vi "Pass State Machine.vi"   [LabVIEW 2013]
uses:
  typedefs/fg_typedef.ctl
  typedefs/subStates.ctl
  typedefs/DevRef Type.ctl
panel:
  # "A State Machine to Handle Passing"
types:
  T1 = typedef "subStates.ctl" = enum16{"null", "wait", "driver control", "auto", "manual override", "hold position", "rotate", "pickup", "pass", "load", "goto shoot", "shoot high goal", "shoot low goal", "cancel arm", "cancel shooter", "end"}
  T2 = typedef "fg_typedef.ctl" = enum16{"Get", "Set"}
  T3 = typedef "DevRef Type.ctl" = enum16{"Shooter Solenoid", "Latch Solenoid", "Right Up Sensor", "Right Down Sensor", "Hold Sensor", "2 Ball Switch", "Arm Encoder"}
  T4 = typedef "WPI_DigitalInputDevRef.ctl" = cluster{"DevStatus":errorcluster, "DIO Channel":T5, "Digital Module":T6}
  T5 = typedef "FPGA_DIOChannel.ctl" = enum8{"DIO 1", "DIO 2", "DIO 3", "DIO 4", "DIO 5", "DIO 6", "DIO 7", "DIO 8", "DIO 9", "DIO 10", "DIO 11", "DIO 12", "DIO 13", "DIO 14", "Invalid"}
  T6 = typedef "FPGA_TypedefDigitalModule.ctl" = enum16{"Digital Module 1", "Digital Module 2"}
  T7 = typedef "WPI_EncoderDevRef.ctl" = cluster{"DevStatus":errorcluster, "EncoderIndex":T8, "CounterIndex":T9, "DistancePerCount":dbl, "Decoding Type":T10}
  T8 = typedef "FPGA_EncoderIdx.ctl" = enum8{"Enc 0", "Enc 1", "Enc 2", "Enc 3", "Invalid"}
  T9 = typedef "FPGA_CounterCtrSystemIndex.ctl" = enum8{"Ctr 0", "Ctr 1", "Ctr 2", "Ctr 3", "Ctr 4", "Ctr 5", "Ctr 6", "Ctr 7", "Invalid"}
  T10 = typedef "WPI_EncoderType.ctl" = enum16{"1x", "2x", "4x"}
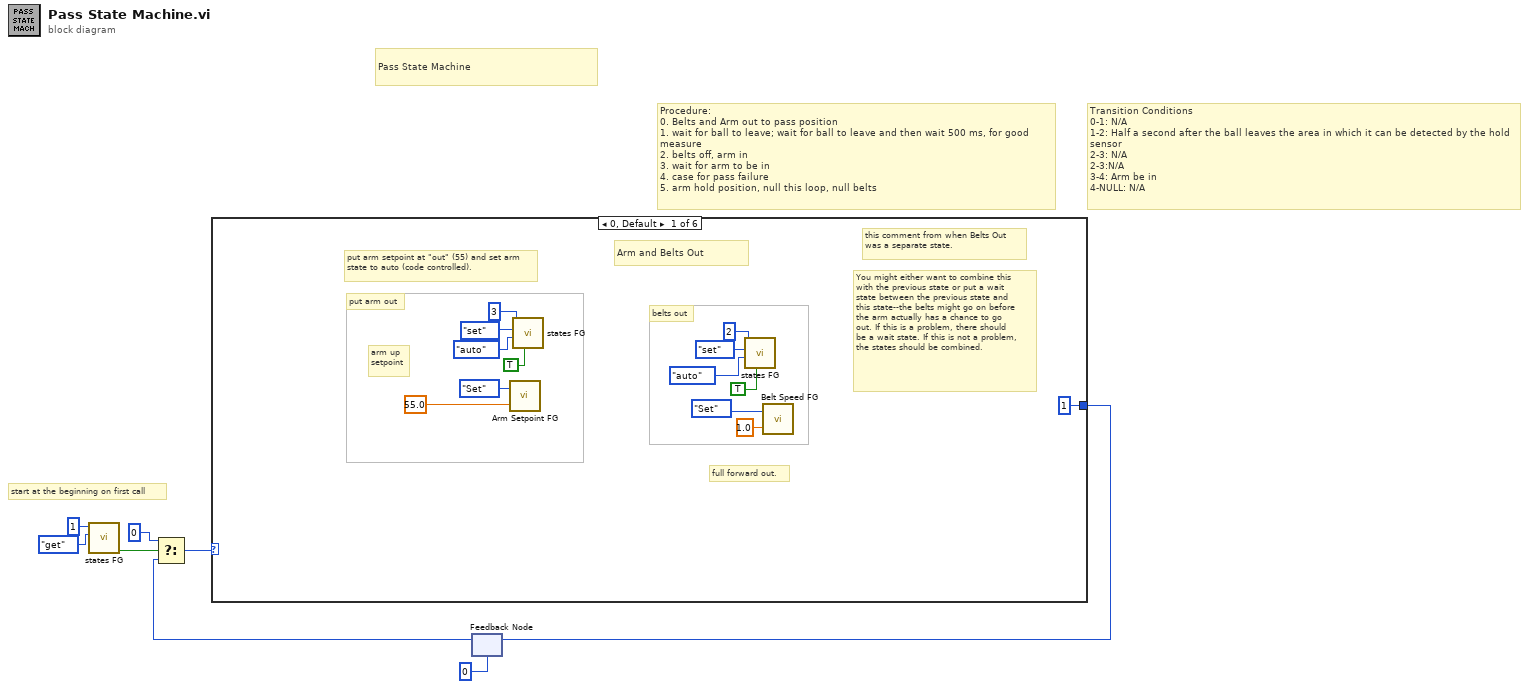
[diagram p0: block diagram]
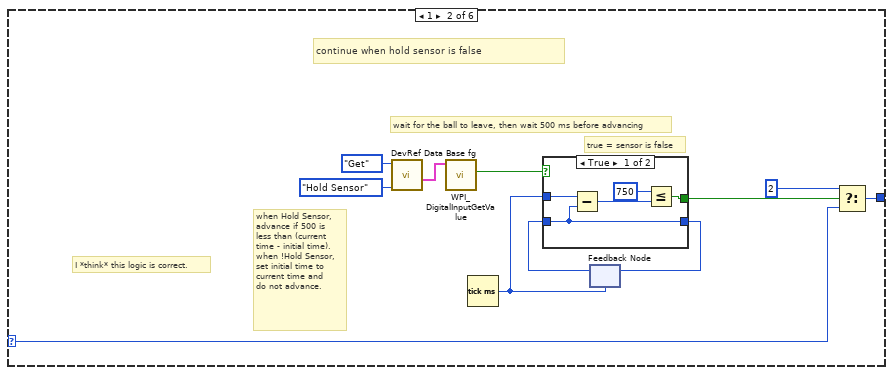
[diagram p2: hidden frame]
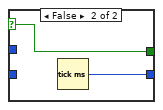
[diagram p3: hidden frame]
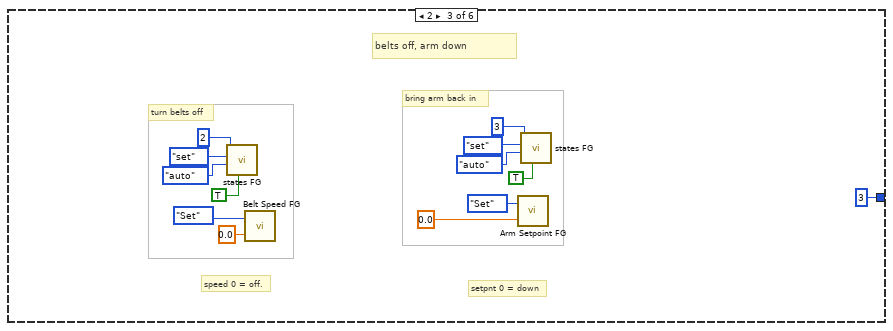
[diagram p4: hidden frame]
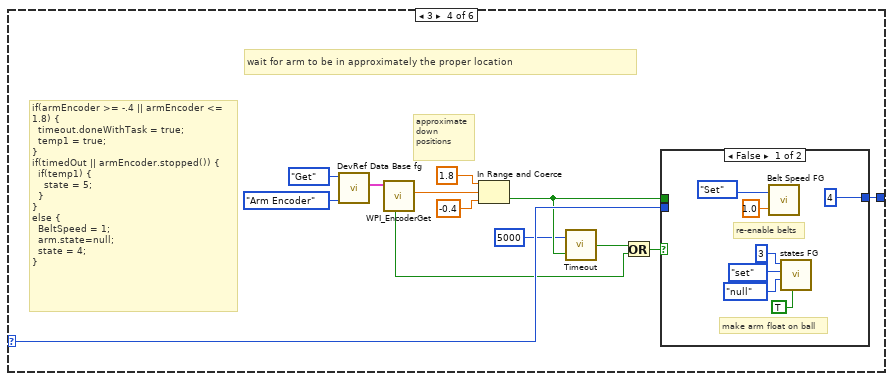
[diagram p5: hidden frame]
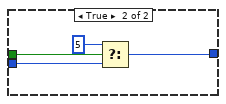
[diagram p6: hidden frame]
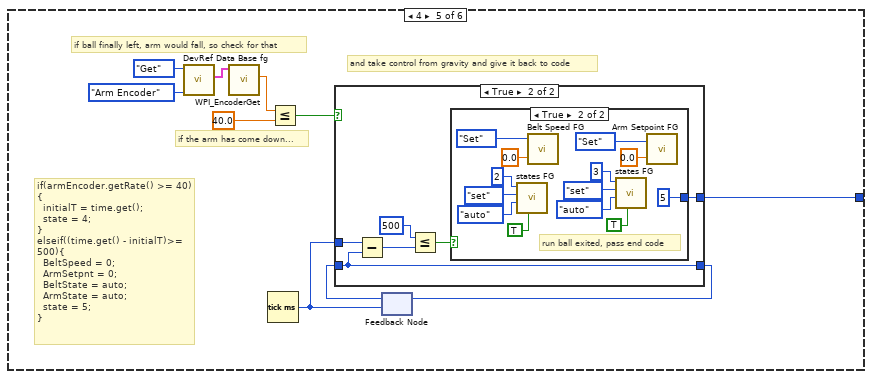
[diagram p7: hidden frame]
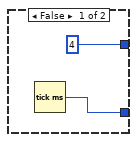
[diagram p8: hidden frame]
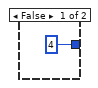
[diagram p9: hidden frame]
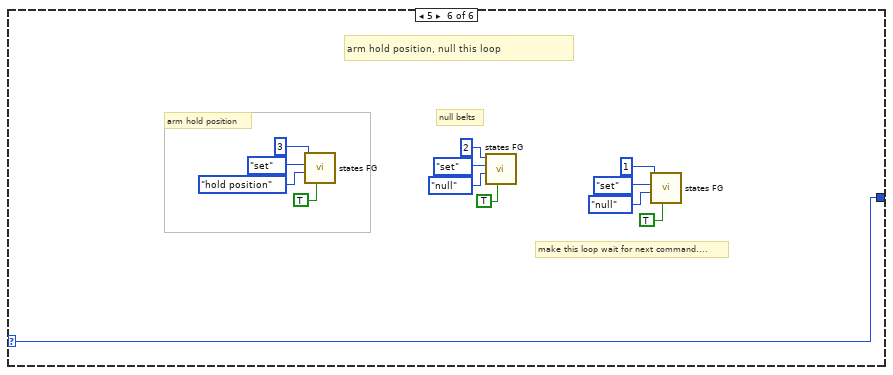
[diagram p10: hidden frame]
diagram:
  # "Transition Conditions\n0-1: N/A\n1-2: Half a second after the ball leaves the area in which it can be detected by the hold sensor\n2-3: N/A\n2-3:N/A\n3-4: Arm be in\n4-NULL: N/A"
  # "Procedure:\n0. Belts and Arm out to pass position\n1. wait for ball to leave; wait for ball to leave and then wait 500 ms, for good measure\n2. belts off, arm in\n3. wait for arm to be in\n4. case for pass failure\n5. arm hold position, null this loop, null belts"
  # "Pass State Machine"
  # "start at the beginning on first call"
  n1 = call "states FG.vi"("menu (get)"=enum16{"set", "get"}."get", "Loop ID"=1) -> ("first call?"=w1:bool)  [unwired: 6 in, 3 out]
  n2 = feedback #1(u8 0) -> (w4:u8)
  n3 = Select(t=u8 0, s=w1, f=w4) -> (s? t:f=w3:u8)
  n4 = case shown="0, Default" w3 {
    selector: w3 -> [_ w28 _ w61 _ w113]
    tunnel: [u8 1 ("t") w27 u8 3 ("t") w60 w78 w113] -> w7
    frame 0, Default {
      # "put arm out"
      # "full forward out."
      # "arm up\nsetpoint"
      # "this comment from when Belts Out\nwas a separate state."
      # "You might either want to combine this\nwith the previous state or put a wait\nstate between the previous state and\nthis state--the belts might go on before\nthe arm actually has a chance to go\nout. If this is a problem, there should\nbe a wait state. If this is not a problem,\nthe states should be combined."
      # "belts out"
      # "put arm setpoint at \"out\" (55) and set arm\nstate to auto (code controlled)."
      # "Arm and Belts Out"
      n5 = call "Arm Setpoint FG.vi"("Setpoint In"=55.0, "Menu"=fg_typedef."Set") -> ()  [unwired: 1 out]
      n6 = call "states FG.vi"("exit in"=TRUE, "subState in"=subStates."auto", "menu (get)"=enum16{"set", "get"}."set", "Loop ID"=3) -> ()  [unwired: 4 in, 4 out]
      n7 = call "states FG.vi"("exit in"=TRUE, "subState in"=subStates."auto", "menu (get)"=enum16{"set", "get"}."set", "Loop ID"=2) -> ()  [unwired: 4 in, 4 out]
      n8 = call "Belt Speed FG.vi"("Speed In"=1.0, "Menu"=fg_typedef."Set") -> ()  [unwired: 1 out]
    }
    frame 1 {
      # "true = sensor is false"
      # "continue when hold sensor is false"
      # "I *think* this logic is correct."
      # "when Hold Sensor,\nadvance if 500 is\nless than (current\ntime - initial time).\nwhen !Hold Sensor,\nset initial time to\ncurrent time and\ndo not advance."
      # "wait for the ball to leave, then wait 500 ms before advancing"
      n9 = call "DevRef Data Base fg.vi"("DevRef to Get"=DevRef_Type."Hold Sensor", "Menu"=fg_typedef."Get") -> ("Selected Sensor"=w29:T4)  [unwired: 2 in, 5 out]
      n10 = call <vilib>:"WPI_DigitalInputGetValue.vi"("DigitalInputDevRef"=w29) -> ("Value"=w23:bool)  [unwired: 8 in, 2 out]
      n11 = Tick Count (ms)() -> (millisecond timer value=w31:u32)
      n12 = feedback #2(w31) -> (w30:u32)
      n13 = case shown="True" w23 {
        selector: w23 -> [_ w38]
        tunnel: [w37 w39] -> w32
        tunnel: w30 -> [w37 _]
        tunnel: w31 -> [w36 _]
        tunnel: [w33 w38] -> w22
        frame True {
          n14 = Subtract(x=w36, y=w37) -> (x-y=w34:u32)
          n15 = Less Or Equal?(x=u32 750, y=w34) -> (x <= y?=w33:bool)
        }
        frame False {
          n16 = Tick Count (ms)() -> (millisecond timer value=w39:u32)
        }
      }
      n17 = feedback-in #2(w32) -> ()
      n18 = Select(t=u8 2, s=w22, f=w28) -> (s? t:f=w27:u8)
    }
    frame 2 {
      # "turn belts off"
      # "bring arm back in"
      # "setpnt 0 = down"
      # "speed 0 = off."
      # "belts off, arm down"
      n19 = call "states FG.vi"("exit in"=TRUE, "subState in"=subStates."auto", "menu (get)"=enum16{"set", "get"}."set", "Loop ID"=2) -> ()  [unwired: 4 in, 4 out]
      n20 = call "Belt Speed FG.vi"("Speed In"=0.0, "Menu"=fg_typedef."Set") -> ()  [unwired: 1 out]
      n21 = call "Arm Setpoint FG.vi"("Setpoint In"=0.0, "Menu"=fg_typedef."Set") -> ()  [unwired: 1 out]
      n22 = call "states FG.vi"("exit in"=TRUE, "subState in"=subStates."auto", "menu (get)"=enum16{"set", "get"}."set", "Loop ID"=3) -> ()  [unwired: 4 in, 4 out]
    }
    frame 3 {
      # "if(armEncoder >= -.4 || armEncoder <= 1.8) {\n  timeout.doneWithTask = true;\n  temp1 = true;\n}\nif(timedOut || armEncoder.stopped()) {\n  if(temp1) {\n    state = 5;\n  }\n}\nelse {\n  BeltSpeed = 1;\n  arm.state=null;\n  state = 4;\n}"
      # "approximate\ndown\npositions"
      # "wait for arm to be in approximately the proper location"
      n23 = call "DevRef Data Base fg.vi"("DevRef to Get"=DevRef_Type."Arm Encoder", "Menu"=fg_typedef."Get") -> ("Selected Encoder"=w65:T7)  [unwired: 2 in, 5 out]
      n24 = call <vilib>:"WPI_EncoderGet.vi"("EncoderDevRef"=w65) -> ("Distance"=w64:dbl, "Stopped"=w53:bool)  [unwired: 5 in, 4 out]
      n25 = In Range and Coerce(upper limit=1.8, x=w64, lower limit=-0.4) -> (In Range?=w57:bool)  [unwired: 1 out]
      n26 = call "Timeout.vi"("Done with Task?"=w57, "Timeout (ms)"=u32 5000) -> ("Timed Out?"=w55:bool)  [unwired: 1 in]
      n27 = Or(x=w55, y=w53) -> (x .or. y?=w54:bool)
      n28 = case shown="False" w54 {
        tunnel: w61 -> [_ w76]
        tunnel: [u8 4 ("t") w75] -> w60
        tunnel: w57 -> [_ w73]
        frame False {
          # "re-enable belts"
          # "make arm float on ball"
          n29 = call "Belt Speed FG.vi"("Speed In"=1.0, "Menu"=fg_typedef."Set") -> ()  [unwired: 1 out]
          n30 = call "states FG.vi"("exit in"=TRUE, "subState in"=subStates."null", "menu (get)"=enum16{"set", "get"}."set", "Loop ID"=3) -> ()  [unwired: 4 in, 4 out]
        }
        frame True {
          n31 = Select(t=u8 5, s=w73, f=w76) -> (s? t:f=w75:u8)
        }
      }
    }
    frame 4 {
      # "if the arm has come down..."
      # "if(armEncoder.getRate() >= 40) {\n  initialT = time.get();\n  state = 4;\n}\nelseif((time.get() - initialT)>= 500){\n  BeltSpeed = 0;\n  ArmSetpnt = 0;\n  BeltState = auto;\n  ArmState = auto;\n  state = 5;\n}"
      # "and take control from gravity and give it back to code"
      # "if ball finally left, arm would fall, so check for that"
      n32 = call "DevRef Data Base fg.vi"("DevRef to Get"=DevRef_Type."Arm Encoder", "Menu"=fg_typedef."Get") -> ("Selected Encoder"=w86:T7)  [unwired: 2 in, 5 out]
      n33 = call <vilib>:"WPI_EncoderGet.vi"("EncoderDevRef"=w86) -> ("Distance"=w77:dbl)  [unwired: 5 in, 5 out]
      n34 = Tick Count (ms)() -> (millisecond timer value=w81:u32)
      n35 = Less Or Equal?(x=w77, y=40.0) -> (x <= y?=w79:bool)
      n36 = feedback #3(w81) -> (w80:u32)
      n37 = case shown="True" w79 {
        tunnel: [w88 w94] -> w82
        tunnel: w80 -> [_ w94]
        tunnel: w81 -> [_ w93]
        tunnel: [u8 4 w89] -> w78
        frame False {
          n38 = Tick Count (ms)() -> (millisecond timer value=w88:u32)
        }
        frame True {
          n39 = Subtract(x=w93, y=w94) -> (x-y=w92:u32)
          n40 = Less Or Equal?(x=u32 500, y=w92) -> (x <= y?=w90:bool)
          n41 = case shown="True" w90 {
            tunnel: [u8 4 u8 5] -> w89
            frame False {
            }
            frame True {
              # "run ball exited, pass end code"
              n42 = call "states FG.vi"("exit in"=TRUE, "subState in"=subStates."auto", "menu (get)"=enum16{"set", "get"}."set", "Loop ID"=2) -> ()  [unwired: 4 in, 4 out]
              n43 = call "Belt Speed FG.vi"("Speed In"=0.0, "Menu"=fg_typedef."Set") -> ()  [unwired: 1 out]
              n44 = call "states FG.vi"("exit in"=TRUE, "subState in"=subStates."auto", "menu (get)"=enum16{"set", "get"}."set", "Loop ID"=3) -> ()  [unwired: 4 in, 4 out]
              n45 = call "Arm Setpoint FG.vi"("Setpoint In"=0.0, "Menu"=fg_typedef."Set") -> ()  [unwired: 1 out]
            }
          }
        }
      }
      n46 = feedback-in #3(w82) -> ()
    }
    frame 5 {
      # "null belts"
      # "arm hold position"
      # "make this loop wait for next command...."
      # "arm hold position, null this loop"
      n47 = call "states FG.vi"("exit in"=TRUE, "subState in"=subStates."hold position", "menu (get)"=enum16{"set", "get"}."set", "Loop ID"=3) -> ()  [unwired: 4 in, 4 out]
      n48 = call "states FG.vi"("exit in"=TRUE, "subState in"=subStates."null", "menu (get)"=enum16{"set", "get"}."set", "Loop ID"=2) -> ()  [unwired: 4 in, 4 out]
      n49 = call "states FG.vi"("exit in"=TRUE, "subState in"=subStates."null", "menu (get)"=enum16{"set", "get"}."set", "Loop ID"=1) -> ()  [unwired: 4 in, 4 out]
    }
  }
  n50 = feedback-in #1(w7) -> ()
